vi "计算长短轴.vi"(0 "灰度图像":T1, 1 "第一点x值，y=0":dbl, 2 "第二点x值，y=479":dbl, 3 "第一点y值，x=0":dbl, 4 "第二点y值，x=639":dbl, 5 "拟合方法":T2 items=["Least Square", "Least Absolute Residual", "Bisquare"], 6 "所在直线 纵":sgl[](array[numeric]), 7 "横纵数组":i32[](array[numeric]), 8 "所在直线 横":sgl[](array[numeric]), 9 "纵轴数组":i32[](array[numeric])) -> (14 "长轴":dbl[][](array[numeric]), 15 "短轴":dbl[][](array[numeric]), 16 "长轴半径um":dbl, 17 "纵轴":dbl[][](array[numeric]), 18 "横轴":dbl[][](array[numeric]), 19 "短轴半径um":dbl)   [LabVIEW 2015]
uses:
  <vilib>/Analysis/6fits.llb/Curve Fitting Criteria.ctl
  <vilib>/vision/Image Controls.llb/IMAQ Image.ctl
  <vilib>/Analysis/NI_AALPro.lvlib
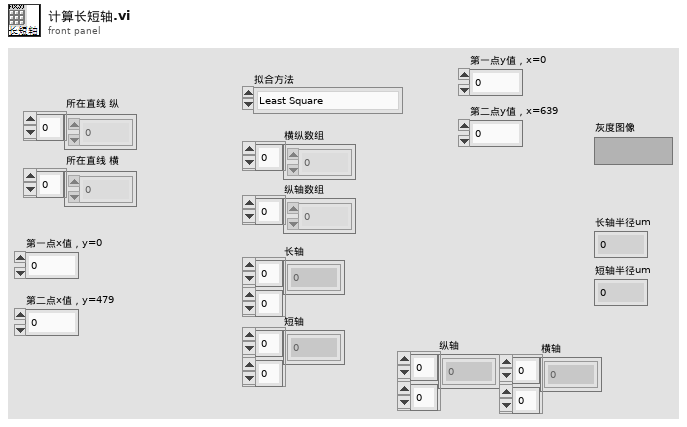
[diagram p1: front panel]
types:
  T1 = typedef "IMAQ Image.ctl" = refnum<image>
  T2 = typedef "NI_AALPro.lvlib/Curve Fitting Criteria.ctl" = u16
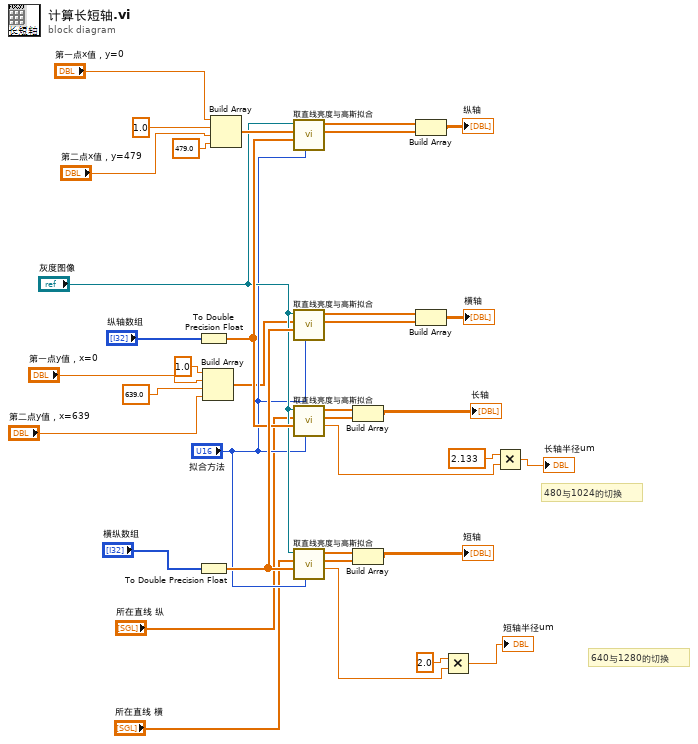
[diagram p0: block diagram]
diagram:
  # "480与1024的切换"
  # "640与1280的切换"
  n1 = To Double Precision Float(number="纵轴数组") -> (double precision float=w27:dbl[])
  n2 = To Double Precision Float(number="横纵数组") -> (double precision float=w28:dbl[])
  n3 = Build Array(1.0, "第一点y值，x=0", 639.0, "第二点y值，x=639") -> (w17:dbl[])
  n4 = Build Array("第一点x值，y=0", 1.0, "第二点x值，y=479", 479.0) -> (w32:dbl[])
  n5 = call "取直线亮度与高斯拟合.vi"("拟合方法"="拟合方法", "X"=w27, "所在直线"=w32, "Image in"="灰度图像") -> ("高斯拟合"=w31:dbl[], "原曲线"=w18:dbl[])  [unwired: 4 in, 2 out]
  n6 = call "取直线亮度与高斯拟合.vi"("拟合方法"="拟合方法", "X"=w28, "所在直线"=w17, "Image in"="灰度图像") -> ("高斯拟合"=w30:dbl[], "原曲线"=w29:dbl[])  [unwired: 4 in, 2 out]
  n7 = call "取直线亮度与高斯拟合.vi"("拟合方法"="拟合方法", "X"=w27, "所在直线"="所在直线 纵", "Image in"="灰度图像") -> ("半径um"=w5:dbl, "高斯拟合"=w21:dbl[], "原曲线"=w22:dbl[])  [unwired: 4 in, 1 out]
  n8 = call "取直线亮度与高斯拟合.vi"("拟合方法"="拟合方法", "X"=w28, "所在直线"="所在直线 横", "Image in"="灰度图像") -> ("半径um"=w2:dbl, "高斯拟合"=w19:dbl[], "原曲线"=w20:dbl[])  [unwired: 4 in, 1 out]
  n9 = Build Array(w22, w21) -> (→"长轴":dbl[][])
  n10 = Build Array(w20, w19) -> (→"短轴":dbl[][])
  n11 = Build Array(w18, w31) -> (→"纵轴":dbl[][])
  n12 = Build Array(w29, w30) -> (→"横轴":dbl[][])
  n13 = Multiply(x=2.0 ("x*y"), y=w2) -> (x*y=→"短轴半径um":dbl)
  n14 = Multiply(x=2.133 ("x*y"), y=w5) -> (x*y=→"长轴半径um":dbl)
